vi "Instrument.sample-registry.getAll.vi"(8 "error in (no error)":errorcluster, 11 "Instrument.sample-registry":refnum<class "Instrument.sample-registry.lvclass">) -> (0 "error out":errorcluster, 2 "getAll":T1, 3 "Instrument.sample-registry out":refnum<class "Instrument.sample-registry.lvclass">)   [LabVIEW 2019, in "Instrument.sample-registry.lvclass"]
uses:
  Instrument.sample-registry.lvclass
  Typedefs/Instrument.sample-registry.getAll--Cluster.ctl
  caf7fc02-a1f0-4077-bb00-48bdf0fcd3b8.vi
  caf7fc02-a1f0-4077-bb00-48bdf0fcd3b8.vi/964b75e0-3056-48cb-9a9a-c477c38c92ec.vi
  caf7fc02-a1f0-4077-bb00-48bdf0fcd3b8.vi/964b75e0-3056-48cb-9a9a-c477c38c92ec.vi/61a8b5a8-0845-438f-a7aa-9e6b14707d81.vi
  caf7fc02-a1f0-4077-bb00-48bdf0fcd3b8.vi/964b75e0-3056-48cb-9a9a-c477c38c92ec.vi/a334a218-ae1a-483a-a8b0-5cbf40bffc95.vi
  caf7fc02-a1f0-4077-bb00-48bdf0fcd3b8.vi/964b75e0-3056-48cb-9a9a-c477c38c92ec.vi/a334a218-ae1a-483a-a8b0-5cbf40bffc95.vi/ff58df35-704e-4df4-b8b6-b4ea359b275b.vi
  caf7fc02-a1f0-4077-bb00-48bdf0fcd3b8.vi/964b75e0-3056-48cb-9a9a-c477c38c92ec.vi/a334a218-ae1a-483a-a8b0-5cbf40bffc95.vi/7a2cf5a1-1432-495d-8ff4-a5b27b143ed7.vi
  <userlib>/LevyLab/Levylab Instruments/SMOs/RemoteControl/API/Remote Client.vi
  <vilib>/JDP Science/JSONtext/JSON text to Variant.vi
  <vilib>/JDP Science/JSONtext/LVClass Serializer/JSONtext LVClass Serializer.lvclass
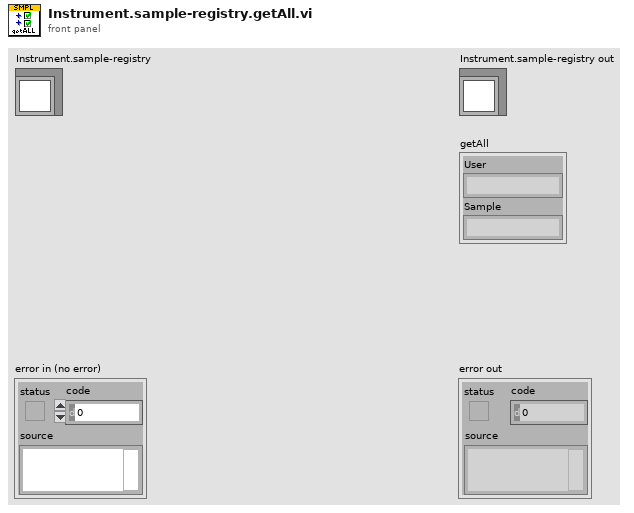
[diagram p1: front panel]
types:
  T1 = typedef "Instrument.sample-registry.lvclass/Instrument.sample-registry.getAll--Cluster.ctl" = cluster{"User":string, "Sample":string}
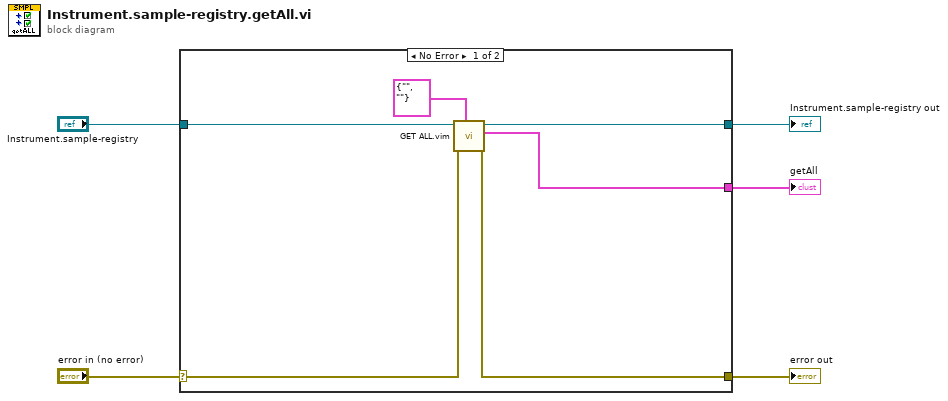
[diagram p0: block diagram]
diagram:
  n1 = case shown="No Error" "error in (no error)" {
    selector: "error in (no error)" -> [w9 w13]
    tunnel: [w8 w13] -> w4
    tunnel: [w10 w12] -> w2
    tunnel: "Instrument.sample-registry" -> [w11 w12]
    tunnel: [w7 _] -> w1
    frame No Error {
      n2 = call "GET ALL.vim"("type"=T1 {"User"="", "Sample"=""} ("getAll"), "error in (no error)"=w9, "Instrument in"=w11) -> ("error out"=w8:errorcluster, "getAll"=w7:T1, "Instrument out"=w10:refnum<class "Instrument.sample-registry.lvclass">)  [unwired: 6 in]
    }
    frame Error {
    }
  }
  "error out" <- w4
  "Instrument.sample-registry out" <- w2
  "getAll" <- w1
